vi "NH485_Test_Globals.vi"() -> ()   [LabVIEW 2014]
panel:
  out "GlobalExit":bool
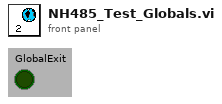
[diagram p1: front panel]
diagram:
